vi "Equalizer.vi"() -> ()   [LabVIEW 2024]
doc: "Use this template to build a producer/consumer design pattern with events to produce queue items. Use this design pattern instead of the User Interface Event Handler pattern for user interfaces when you want to execute code asynchronously in response to an event without slowing the user interface responsiveness."
uses:
  <vilib>/sound2/lvsound2.llb/Sound Data Format.ctl
  <vilib>/sound2/lvsound2.llb/Sampling Mode.ctl
  <vilib>/sound2/lvsound2.llb/Sound Input Read (DBL).vi
  <vilib>/measure/maspectr.llb/FFT Spectrum (Mag-Phase) for 1 Chan.vi
  <vilib>/sound2/lvsound2.llb/Sound Output Write (DBL Single).vi
  <vilib>/measure/NI_MAPro.lvlib
panel:
  out "Modified Speech - spectrum":cluster{"f0":dbl, "df":dbl, "magnitude":dbl[]}(graph)
  out "Modified Speech":waveform(dbl)(graph)
  out "Original speech":waveform(dbl)[](graph)
  out "Boolean":bool
  in  "Save To File 2":bool
  in  "Treble":dbl(slide)=1.0 scale=0.0..1.0
  in  "Mid":dbl(slide)=1.0 scale=0.0..1.0
  in  "Bass":dbl(slide)=1.0 scale=0.0..1.0
  in  "Pitch changer":dbl(slide)=1.0459183673469388 scale=0.3..2.0
  in  "Modified Voice Volume":dbl(slide)=1.0204081632653061 scale=0.0..10.0
  in  "sound format":T1={"sample rate (S/s)"=44100.0, "number of channels"=2, "bits per sample"=16}
  in  "Start Recording":bool
  # "Equalizer for Microphone"
  # "Voice Volume"
  # "Changing Pitch"
  # "Tones Modification"
  # "Record your voice"
  # "Save to File"
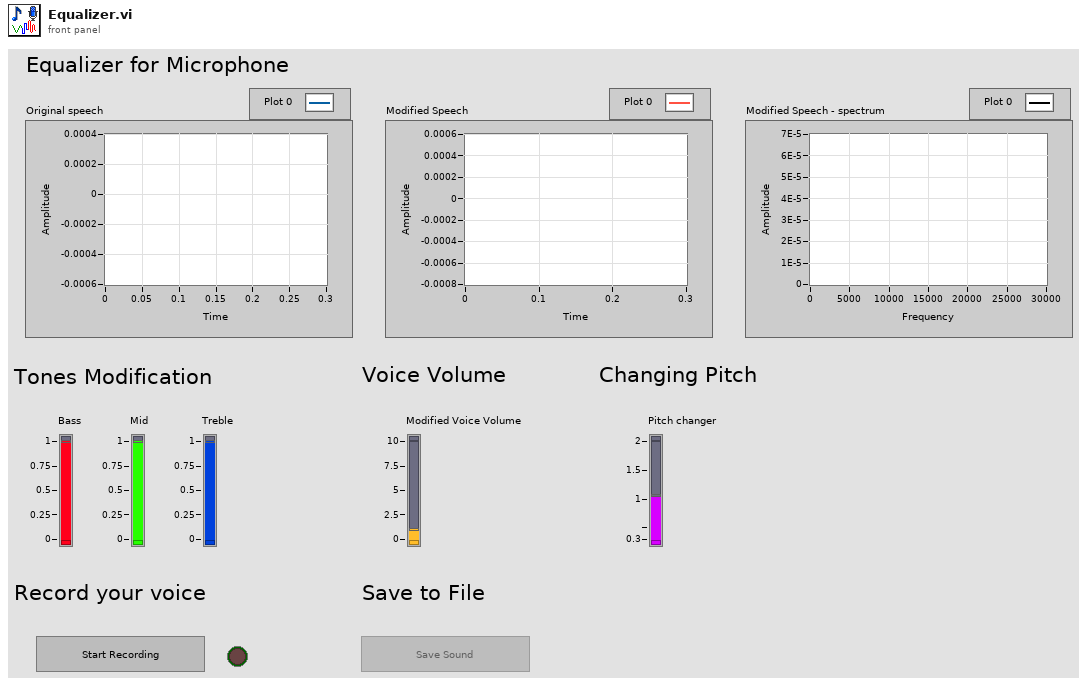
[diagram p1: front panel]
types:
  T1 = typedef "Sound Data Format.ctl" = cluster{"sample rate (S/s)":dbl, "number of channels":i32, "bits per sample":i32}
  T2 = typedef "Sampling Mode.ctl" = i32
  T3 = typedef "Sound Output Task ID.ctl" = u32
  T4 = typedef "Sound Input Task ID.ctl" = u32
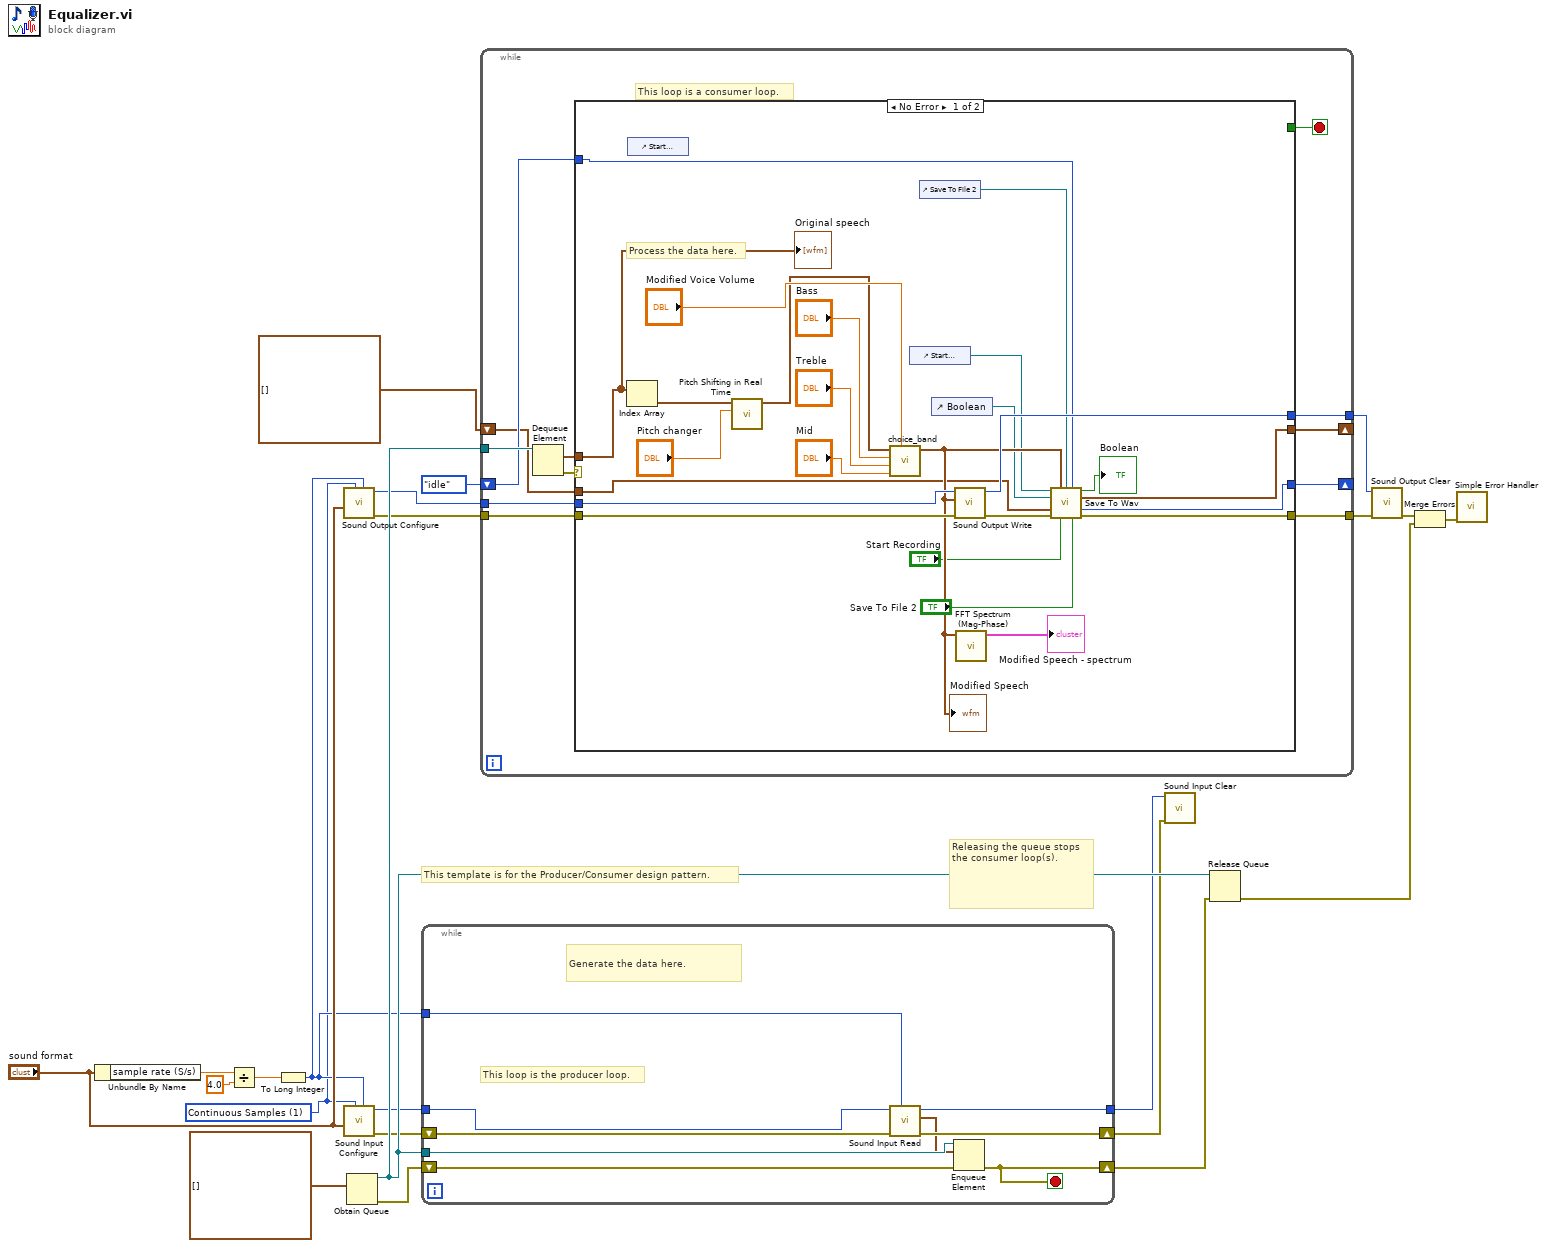
[diagram p0: block diagram]
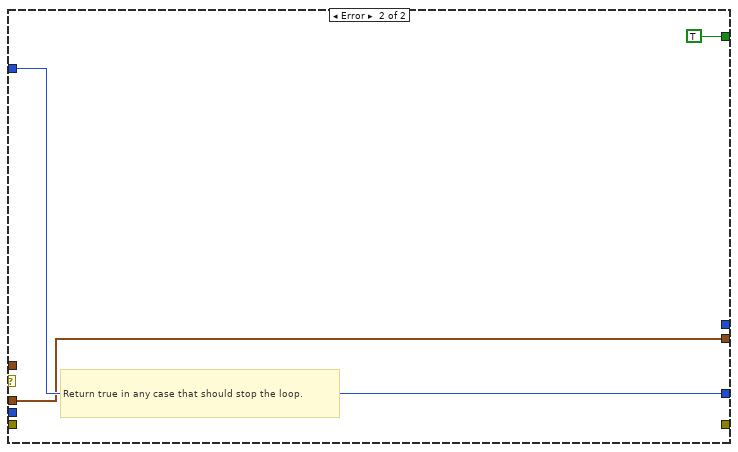
[diagram p2: hidden frame]
diagram:
  w8 = T2 1 items=["Finite Samples", "Continuous Samples"] ("sample mode")
  # "Releasing the queue stops the consumer loop(s)."
  # "This template is for the Producer/Consumer design pattern."
  n1 = Unbundle By Name("sound format") -> ("sample rate (S/s)"=w19:dbl)
  n2 = Divide(x=w19, y=4.0) -> (x/y=w17:dbl)
  n3 = To Long Integer(number=w17) -> (32bit integer=w9:i32)
  n4 = call <vilib>:"Sound Output Configure.vi"("number of samples/ch"=w9, "sample mode"=w8, "sound format"="sound format") -> ("error out"=w11:errorcluster, "task ID"=w12:T3)  [unwired: 7 in]
  n5 = call <vilib>:"Sound Input Configure.vi"("number of samples/ch"=w9, "sample mode"=w8, "sound format"="sound format") -> ("error out"=w15:errorcluster, "task ID"=w16:T4)  [unwired: 7 in]
  n6 = Obtain Queue(element data type=waveform(dbl)[] [] ("data")) -> (queue out=w21:refnum<queue>, error out=w23:errorcluster)  [unwired: 4 in, 1 out]
  n7 = while {
    shift-right: [w24] -> w22
    shift-left: w23 -> [w31]
    tunnel: w21 -> [w32]
    tunnel: w16 -> [w30]
    tunnel: [w27] -> w13
    tunnel: w9 -> [w26]
    shift-right: [w28] -> w14
    shift-left: w15 -> [w29]
    stop <- w24 stop-if-true
    # "Generate the data here."
    # "This loop is the producer loop."
    n8 = call-poly <vilib>:"Sound Input Read.vi"("number of samples/ch"=w26, "error in (no error)"=w29, "task ID"=w30) -> ("error out"=w28:errorcluster, "data"=w25:waveform(dbl)[], "task ID out"=w27:T4)  [unwired: 6 in]
    n9 = Enqueue Element(queue=w32, element=w25, error in (no error)=w31) -> (error out=w24:errorcluster)  [unwired: 1 in, 2 out]
  }
  n10 = while {
    tunnel: w21 -> [w44]
    tunnel: w12 -> [w40]
    tunnel: w11 -> [w39]
    tunnel: [w38] -> w7
    tunnel: [w37] -> w6
    shift-right: [w36] -> _
    shift-left: enum16{"idle", "open", "write", "save"}."idle" -> [w35]
    shift-right: [w34] -> _
    shift-left: waveform(dbl)[] [] -> [w33]
    stop <- w41 stop-if-true
    # "This loop is a consumer loop."
    n11 = Dequeue Element(queue=w44) -> (element=w42:waveform(dbl)[], error out=w43:errorcluster)  [unwired: 2 in, 2 out]
    n12 = case shown="No Error" w43 {
      tunnel: w42 -> [w59 _]
      tunnel: [_ TRUE] -> w41
      tunnel: w40 -> [w69 _]
      tunnel: w39 -> [w68 _]
      tunnel: [w67 _] -> w38
      tunnel: [w52 _] -> w37
      tunnel: [w45 w71] -> w36
      tunnel: w35 -> [w55 w71]
      tunnel: [w46 w70] -> w34
      tunnel: w33 -> [w54 w70]
      frame No Error {
        # "Process the data here."
        n13 = Index Array(array=w59) -> (element=w66:waveform(dbl))  [unwired: 1 in]
        n14 = control-ref of="Start Recording"() -> ()  [unwired: 1 out]
        n15 = call "Pitch Shifting in Real Time.vi"("Pitch multiplier"="Pitch changer", "output waveform 2"=w66) -> ("output waveform"=w60:waveform(dbl))  [unwired: 5 in, 2 out]
        n16 = call "choice_band.vi"("Master Volume"="Modified Voice Volume", "Mid tone"="Mid", "Treble"="Treble", "Bass"="Bass", "input waveform"=w60) -> ("output waveform"=w57:waveform(dbl))  [unwired: 6 in]
        "Modified Speech" <- w57
        n17 = control-ref of="Start Recording"() -> (w49:refnum<vi>)
        n18 = control-ref of="Save To File 2"() -> (w56:refnum<vi>)
        n19 = control-ref of="Boolean"() -> (w48:refnum<vi>)
        n20 = call-poly <vilib>:"Sound Output Write.vi"("error in (no error)"=w68, "data"=w57, "task ID"=w69) -> ("error out"=w53:errorcluster, "task ID out"=w67:T3)  [unwired: 7 in]
        n21 = call-poly <vilib>:"FFT Spectrum (Mag-Phase).vi"("time signal"=w57) -> ("magnitude"=→"Modified Speech - spectrum":cluster{"f0":dbl, "df":dbl, "magnitude":dbl[]})  [unwired: 6 in, 4 out]
        n22 = call "Save To Wav.vi"("Boolean in"=w49, "output waveform"=w57, "Bool Refnum"=w56, "Enum in"=w55, "reference in"=w48, "Array in"=w54, "error in (no error)"=w53, "Start Recording"="Start Recording", "Save To File in"="Save To File 2") -> ("Boolean"=→"Boolean":bool, "Array out"=w46:waveform(dbl)[], "Enum out"=w45:enum16{"idle", "open", "write", "save"}, "error out"=w52:errorcluster)  [unwired: 3 in]
        "Original speech" <- w59
      }
      frame Error {
        # "Return true in any case that should stop the loop."
      }
    }
  }
  n23 = call <vilib>:"Sound Input Clear.vi"("error in (no error)"=w14, "task ID"=w13) -> ()  [unwired: 9 in, 1 out]
  n24 = Release Queue(queue=w21, error in (no error)=w22) -> (error out=w2:errorcluster)  [unwired: 1 in, 2 out]
  n25 = call <vilib>:"Sound Output Clear.vi"("error in (no error)"=w6, "task ID"=w7) -> ("error out"=w3:errorcluster)  [unwired: 9 in]
  n26 = Merge Errors(w3, w2) -> (w1:errorcluster)
  n27 = call <vilib>:"Simple Error Handler.vi"("error in (no error)"=w1) -> ()  [unwired: 4 in, 5 out]
